vi "test Multi FPGA.vi"(8 "error in (no error)":errorcluster, 11 "TestCase in":refnum<class "Mutation Test Case.lvclass">) -> (0 "error out":errorcluster, 3 "TestCase out":refnum<class "Mutation Test Case.lvclass">)   [LabVIEW 2015, in "Mutation Test Case.lvclass"]
uses:
  Mutation Test Case.lvclass
  Shared/Properties.vi
  Shared/Constants and GUIDs.vi
  <vilib>/NI Veristand/Custom Device API/Get Item Property (String Array).vi
  <vilib>/NI Veristand/Custom Device Tools/Custom Device Utility Library/NI VeriStand - Search for All Items by GUID.vi
  <vilib>/NI Veristand/Custom Device API/Get Item Property (String).vi
  <vilib>/addons/_JKI Toolkits/VI Tester/TestCase.llb/TestCase.lvclass
  System Explorer/Engine Simulation Toolkit System Explorer.lvlib
  <vilib>/NI VeriStand/Custom Device API/Custom Device API.lvlib
  Shared/Engine Simulation Toolkit Shared.lvlib
  <vilib>/NI VeriStand/Custom Device Tools/Custom Device Utility Library/Custom Device Utility Library.lvlib
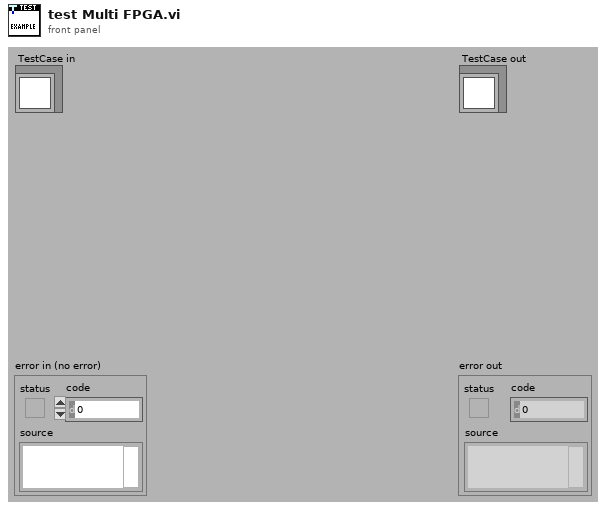
[diagram p1: front panel]
types:
  T1 = typedef "Custom Device API.lvlib/Custom Device Item Ref.ctl" = u64
  T2 = typedef "Custom Device API.lvlib/Custom Device Item Info.ctl" = cluster{"Name":string, "Is Channel":bool, "GUID":string, "Is Waveform":bool}
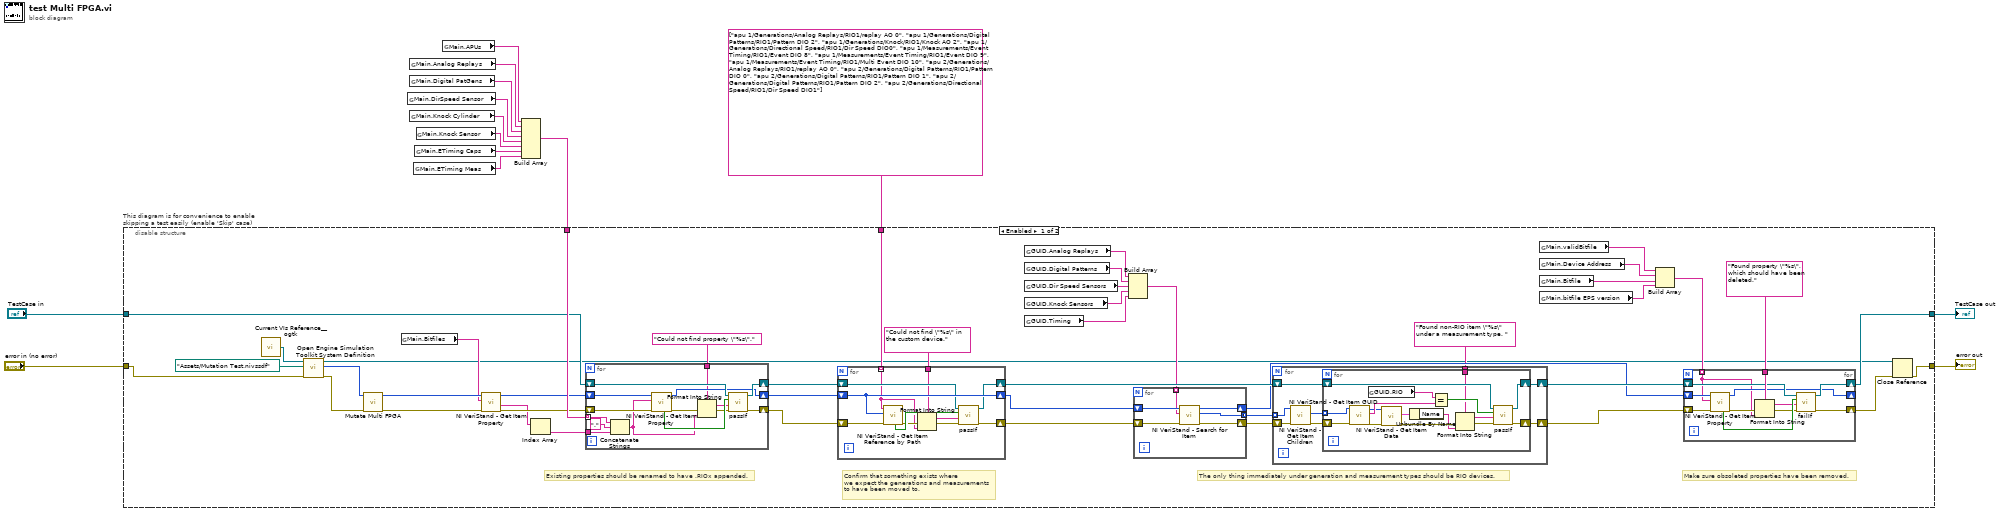
[diagram p0: block diagram]
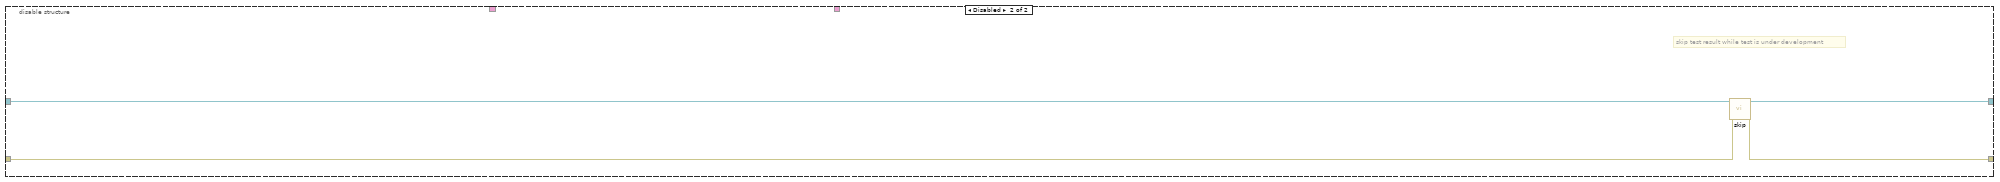
[diagram p2: hidden frame]
diagram:
  n1 = global read "Properties.vi" "Main.DirSpeed Sensor"() -> (w6:string)
  n2 = global read "Properties.vi" "Main.Analog Replays"() -> (w4:string)
  n3 = global read "Properties.vi" "Main.Digital PatGens"() -> (w5:string)
  n4 = global read "Properties.vi" "Main.Knock Cylinder"() -> (w7:string)
  n5 = global read "Properties.vi" "Main.ETiming Meas"() -> (w9:string)
  n6 = global read "Properties.vi" "Main.ETiming Caps"() -> (w8:string)
  n7 = global read "Properties.vi" "Main.Knock Sensor"() -> (w10:string)
  n8 = global read "Properties.vi" "Main.APUs"() -> (w3:string)
  n9 = Build Array(w3, w4, w5, w6, w7, w10, w8, w9) -> (w2:string[])
  n10 = disable-structure "This diagram is for convenience to enable skipping a test easily (enable 'Skip' case)" shown="Enabled" {
    disable-tunnel: "TestCase in" -> [w18 w131]
    disable-tunnel: [w48 w129] -> w12
    disable-tunnel: [w46 w130] -> w1
    disable-tunnel: "error in (no error)" -> [w57 w128]
    disable-tunnel: string[] ["apu 1/Generations/Analog Replays/RIO1/replay AO 0", "apu 1/Generations/Digital Patterns/RIO1/Pattern DIO 2", "apu 1/Generations/Knock/RIO1/Knock AO 2", "apu 1/Generations/Directional Speed/RIO1/Dir Speed DIO0", "apu 1/Measurements/Event Timing/RIO1/Event DIO 8", "apu 1/Measurements/Event Timing/RIO1/Event DIO 9", "apu 1/Measurements/Event Timing/RIO1/Multi Event DIO 10", "apu 2/Generations/Analog Replays/RIO1/replay AO 0", "apu 2/Generations/Digital Patterns/RIO1/Pattern DIO 0", "apu 2/Generations/Digital Patterns/RIO1/Pattern DIO 1", "apu 2/Generations/Digital Patterns/RIO1/Pattern DIO 2", "apu 2/Generations/Directional Speed/RIO1/Dir Speed DIO1"] ("string array") -> [w45 _]
    disable-tunnel: w2 -> [w26 _]
    frame Enabled {
      # "Existing properties should be renamed to have .RIOx appended."
      # "Make sure obsoleted properties have been removed."
      # "The only thing immediately under generation and measurement types should be RIO devices."
      # "Confirm that something exists where\nwe expect the generations and measurements\nto have been moved to."
      n11 = call <userlib>:"Current VIs Reference__ogtk.vi"() -> ("Current VI's reference"=w59:refnum<vi>)  [unwired: 5 in]
      n12 = call "Open Engine Simulation Toolkit System Definition.vi"("error in (no error)"=w57, "System Definition Path"=path "Assets/Mutation Test.nivssdf" ("Absolute or Relative Path"), "Current VI in"=w59) -> ("error out"=w47:errorcluster, "Engine Simulation Toolkit NodeID"=w56:u64, "SystemDefinition"=w16:refnum<k24>)  [unwired: 6 in]
      n13 = call "Mutate Multi FPGA.vi"("error in (no error)"=w47, "Device Ref in"=w56) -> ("error out"=w15:errorcluster, "Device Ref out"=w25:T1)  [unwired: 8 in]
      n14 = global read "Properties.vi" "Main.Bitfiles"() -> (w22:string)
      n15 = call-poly <vilib>:"NI VeriStand - Get Item Property.vi"("error in (no error)"=w15, "Property Name"=w22, "Item Ref in"=w25) -> ("error out"=w24:errorcluster, "Value"=w21:string[], "Item Ref out"=w23:T1)  [unwired: 5 in, 1 out]
      n16 = Index Array(array=w21) -> (element=w20:string)  [unwired: 1 in]
      n17 = for {
        tunnel: w26 -> [w73] mode=indexing
        shift-right: [w69] -> w28
        shift-left: w24 -> [w71]
        shift-right: [w66] -> w27
        shift-left: w23 -> [w70]
        tunnel: w20 -> [w72]
        shift-right: [w67] -> w19
        shift-left: w18 -> [w68]
        tunnel: "Could not find property \"%s\"." ("format string") -> [w60]
        n18 = Concatenate Strings(w73, "." ("string"), w72) -> (w61:string)
        n19 = call-poly <vilib>:"NI VeriStand - Get Item Property.vi"("error in (no error)"=w71, "Property Name"=w61, "Item Ref in"=w70) -> ("error out"=w64:errorcluster, "Item Ref out"=w66:T1, "Found?"=w65:bool)  [unwired: 5 in, 1 out]
        n20 = Format Into String(format string=w60, error in=w64, w61) -> (resulting string=w62:string, error out=w63:errorcluster)  [unwired: 1 in]
        n21 = call-dynamic "passIf.vi"("error in (no error)"=w63, "message (\"\")"=w62, "pass"=w65, "TestCase in"=w68) -> ("error out"=w69:errorcluster, "TestCase out"=w67:refnum<class "Mutation Test Case.lvclass">)  [unwired: 6 in]
      }
      n22 = for {
        shift-right: [w82] -> w40
        shift-left: w28 -> [w84]
        shift-right: [w85] -> w37
        shift-left: w27 -> [w85]
        tunnel: w45 -> [w76] mode=indexing
        shift-right: [w80] -> w42
        shift-left: w19 -> [w81]
        tunnel: "Could not find \"%s\" in the custom device." ("format string") -> [w75]
        n23 = call <vilib>:"NI VeriStand - Get Item Reference by Path.vi"("error in (no error)"=w84, "Root Ref"=w85, "Item Path in"=w76) -> ("error out"=w79:errorcluster, "Found"=w83:bool)  [unwired: 5 in, 2 out]
        n24 = Format Into String(format string=w75, error in=w79, w76) -> (resulting string=w77:string, error out=w78:errorcluster)  [unwired: 1 in]
        n25 = call-dynamic "passIf.vi"("error in (no error)"=w78, "message (\"\")"=w77, "pass"=w83, "TestCase in"=w81) -> ("error out"=w82:errorcluster, "TestCase out"=w80:refnum<class "Mutation Test Case.lvclass">)  [unwired: 6 in]
      }
      n26 = global read "Constants and GUIDs.vi" "GUID.Analog Replays"() -> (w30:string)
      n27 = global read "Constants and GUIDs.vi" "GUID.Digital Patterns"() -> (w31:string)
      n28 = global read "Constants and GUIDs.vi" "GUID.Dir Speed Sensors"() -> (w32:string)
      n29 = global read "Constants and GUIDs.vi" "GUID.Knock Sensors"() -> (w33:string)
      n30 = global read "Constants and GUIDs.vi" "GUID.Timing"() -> (w34:string)
      n31 = Build Array(w30, w31, w32, w33, w34) -> (w29:string[])
      n32 = for {
        tunnel: [w89] -> w38 mode=concatenating
        shift-right: [w90] -> w39
        shift-left: w40 -> [w91]
        shift-right: [w87] -> w36
        shift-left: w37 -> [w88]
        tunnel: w29 -> [w86] mode=indexing
        n33 = call-poly <vilib>:"NI VeriStand - Search for Item.vi"("error in"=w91, "Item GUID"=w86, "Section Ref in"=w88) -> ("error out"=w90:errorcluster, "Item Refs"=w89:T1[], "Section Ref out"=w87:T1)  [unwired: 5 in, 1 out]
      }
      n34 = for {
        shift-right: [w97] -> w41
        shift-left: w42 -> [w96]
        shift-right: [w95] -> w43
        shift-left: w39 -> [w94]
        tunnel: w38 -> [w93] mode=indexing
        tunnel: "Found non-RIO item \"%s\" under a measurement type. " ("format string") -> [w92]
        n35 = call <vilib>:"NI VeriStand - Get Item Children.vi"("error in (no error)"=w94, "Item Ref in"=w93) -> ("error out"=w99:errorcluster, "Child Refs"=w98:T1[])  [unwired: 6 in, 2 out]
        n36 = for {
          shift-right: [w115] -> w95
          shift-left: w99 -> [w113]
          tunnel: w98 -> [w111] mode=indexing
          shift-right: [w110] -> w97
          shift-left: w96 -> [w109]
          tunnel: w92 -> [w105]
          n37 = call <vilib>:"NI VeriStand - Get Item GUID.vi"("error in (no error)"=w113, "Item Ref in"=w111) -> ("error out"=w104:errorcluster, "GUID"=w114:string, "Item Ref out"=w103:T1)  [unwired: 7 in]
          n38 = global read "Constants and GUIDs.vi" "GUID.RIO"() -> (w108:string)
          n39 = call <vilib>:"NI VeriStand - Get Item Data.vi"("error in (no error)"=w104, "Item Ref in"=w103) -> ("error out"=w101:errorcluster, "Item Info"=w102:T2)  [unwired: 6 in, 2 out]
          n40 = Unbundle By Name(w102) -> ("Name"=w100:string)
          n41 = Equal?(x=w108, y=w114) -> (x = y?=w112:bool)
          n42 = Format Into String(format string=w105, error in=w101, w100) -> (resulting string=w106:string, error out=w107:errorcluster)  [unwired: 1 in]
          n43 = call-dynamic "passIf.vi"("error in (no error)"=w107, "message (\"\")"=w106, "pass"=w112, "TestCase in"=w109) -> ("error out"=w115:errorcluster, "TestCase out"=w110:refnum<class "Mutation Test Case.lvclass">)  [unwired: 6 in]
        }
      }
      n44 = global read "Properties.vi" "Main.validBitfile"() -> (w54:string)
      n45 = global read "Properties.vi" "Main.Device Address"() -> (w55:string)
      n46 = global read "Properties.vi" "Main.Bitfile"() -> (w53:string)
      n47 = global read "Properties.vi" "Main.bitfile EPS version"() -> (w52:string)
      n48 = Build Array(w54, w55, w53, w52) -> (w51:string[])
      n49 = for {
        shift-right: [w123] -> w49
        shift-left: w43 -> [w126]
        shift-right: [w124] -> w48
        shift-left: w41 -> [w121]
        tunnel: w51 -> [w116] mode=indexing
        tunnel: "Found property \"%s\", which should have been deleted." ("format string") -> [w122]
        shift-right: [w117] -> _
        shift-left: w36 -> [w127]
        n50 = call-poly <vilib>:"NI VeriStand - Get Item Property.vi"("error in (no error)"=w126, "Property Name"=w116, "Item Ref in"=w127) -> ("error out"=w120:errorcluster, "Item Ref out"=w117:T1, "Found?"=w125:bool)  [unwired: 5 in, 1 out]
        n51 = Format Into String(format string=w122, error in=w120, w116) -> (resulting string=w118:string, error out=w119:errorcluster)  [unwired: 1 in]
        n52 = call-dynamic "failIf.vi"("error in (no error)"=w119, "message (\"\")"=w118, "fail"=w125, "TestCase in"=w121) -> ("error out"=w123:errorcluster, "TestCase out"=w124:refnum<class "Mutation Test Case.lvclass">)  [unwired: 6 in]
      }
      n53 = Close Reference(reference=w16, error in (no error)=w49) -> (error out=w46:errorcluster)
    }
    frame Disabled {
      # "skip test result while test is under development"
      n54 = call <vilib>:"skip.vi"("error in (no error)"=w128, "TestCase in"=w131) -> ("error out"=w130:errorcluster, "TestCase out"=w129:refnum<class "Mutation Test Case.lvclass">)  [unwired: 8 in]
    }
  }
  "error out" <- w1
  "TestCase out" <- w12
